vi "Helper SubVI - Generate Chirplet Parameters.vi"(9 "# of sigma (3.5)":dbl=3.5 format="%.2f", 10 "test conditions":T3 {"Sonic Speed [m/s]" format="%.2f"; "Sample Rate [Hz]" format="%.2f"}, 11 "chirplet settings":T2 {"Chirplet Length [m]" format="%.2f"; "Bandwidth [Hz]" format="%.2f"; "F Central [Hz]" format="%.2f"}) -> (3 "chirplet parameters":T1={"alpha"=0.005, "t0"=100.0, "omega"=0.6, "beta"=0.01} {"beta" step=0.0001 format="%.2e"; "omega" format="%.2e"; "t0" format="%.3e"; "alpha" format="%.2e"})   [LabVIEW 2023]
doc: "Generates Chirplet parameters including t0, alpha, beta and omega."
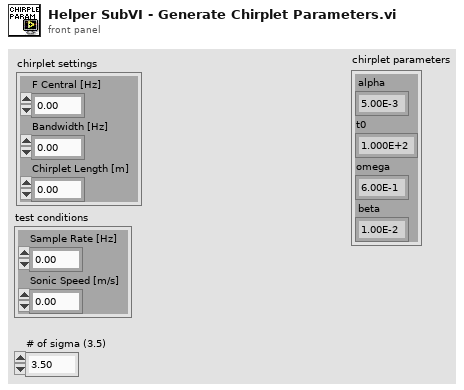
[diagram p1: front panel]
types:
  T1 = cluster{"alpha":dbl, "t0":dbl, "omega":dbl, "beta":dbl}
  T2 = cluster{"F Central [Hz]":dbl, "Bandwidth [Hz]":dbl, "Chirplet Length [m]":dbl}
  T3 = cluster{"Sample Rate [Hz]":dbl, "Sonic Speed [m/s]":dbl}
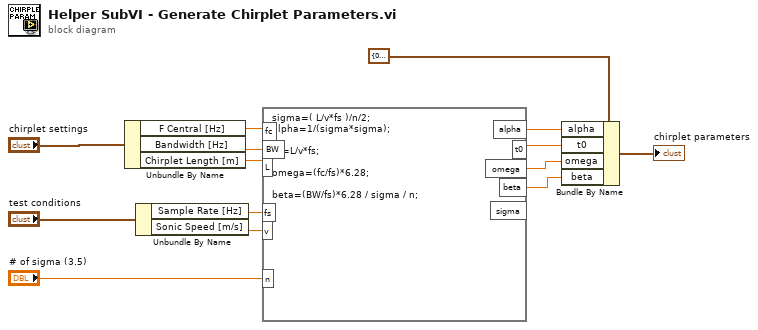
[diagram p0: block diagram]
diagram:
  n1 = Unbundle By Name("chirplet settings") -> ("F Central [Hz]"=w10:dbl, "Bandwidth [Hz]"=w9:dbl, "Chirplet Length [m]"=w8:dbl)
  n2 = Unbundle By Name("test conditions") -> ("Sample Rate [Hz]"=w7:dbl, "Sonic Speed [m/s]"=w6:dbl)
  n3 = formula code="sigma=( L/v*fs )/n/2;\nalpha=1/(sigma*sigma);\n\nt0=L/v*fs;\n\nomega=(fc/fs)*6.28;\n\nbeta=(BW/fs)*6.28 / sigma / n;"("fc"=w10, "BW"=w9, "L"=w8, "fs"=w7, "v"=w6, "n"="# of sigma (3.5)") -> ("alpha"=w4:dbl, "omega"=w2:dbl, "beta"=w3:dbl, "t0"=w1:dbl)  [unwired: 1 out]
  n4 = Bundle By Name(cluster=T1 {"alpha"=0.005, "t0"=100.0, "omega"=0.6, "beta"=0.01} ("chirplet parameters"), "alpha"=w4, "t0"=w1, "omega"=w2, "beta"=w3) -> (→"chirplet parameters":T1)
